vi "DHE_StartTPNT.vi"(8 "error in (no error)":errorcluster) -> (0 "error out":errorcluster)   [LabVIEW 2016]
panel:
  in  "VI path":path=path "/home/ArcVIEW/Modules/TPNT/public/vis"
  in  "VI name":string="TPNT_Main.vi"
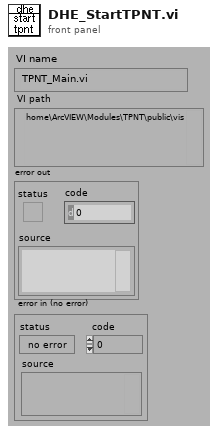
[diagram p1: front panel]
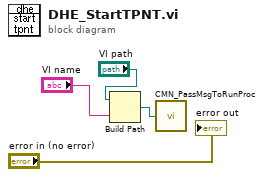
[diagram p0: block diagram]
diagram:
  n1 = Build Path(base path="VI path", name or relative path="VI name") -> (appended path=w1:path)
  n2 = call "CMN_PassMsgToRunProc.vi"("VItoRun"=w1) -> ()  [unwired: 2 in, 13 out]
  "error out" <- "error in (no error)"
